vi "pretank.vi"() -> ()   [LabVIEW 2018]
panel:
  in  "stop":bool
  out "Running":bool
  out "String":string
  out "Cup\nFilling":bool
  out "Heater":bool
  out "Belt":bool
  out "Pump":bool
  out "Temperture":dbl(slide) scale=0.0..100.0
  out "TANK":dbl(slide) scale=0.0..10.0
  in  "Temp preset Value":dbl
  in  "Tank Preset Value":dbl
  in  "Heat Tank":dbl
  in  "Fill Tank":dbl
  in  "Reset":bool
  in  "Sensor 2":bool
  in  "Sensor 1":bool
  in  "Start":bool
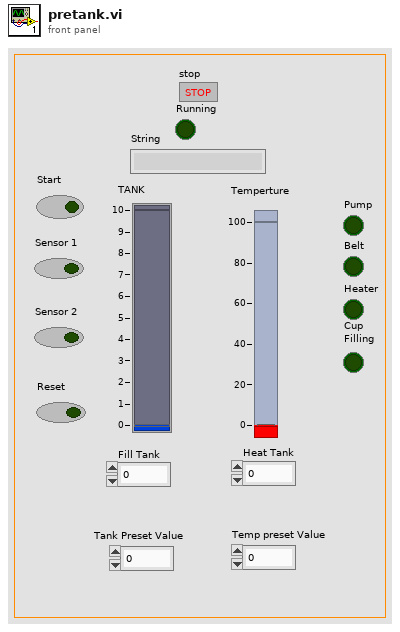
[diagram p1: front panel]
types:
  T1 = enum16{"Start", "Fill", "Sensor 1", "Heat", "Cup", "Sensor 2", "OFF"}
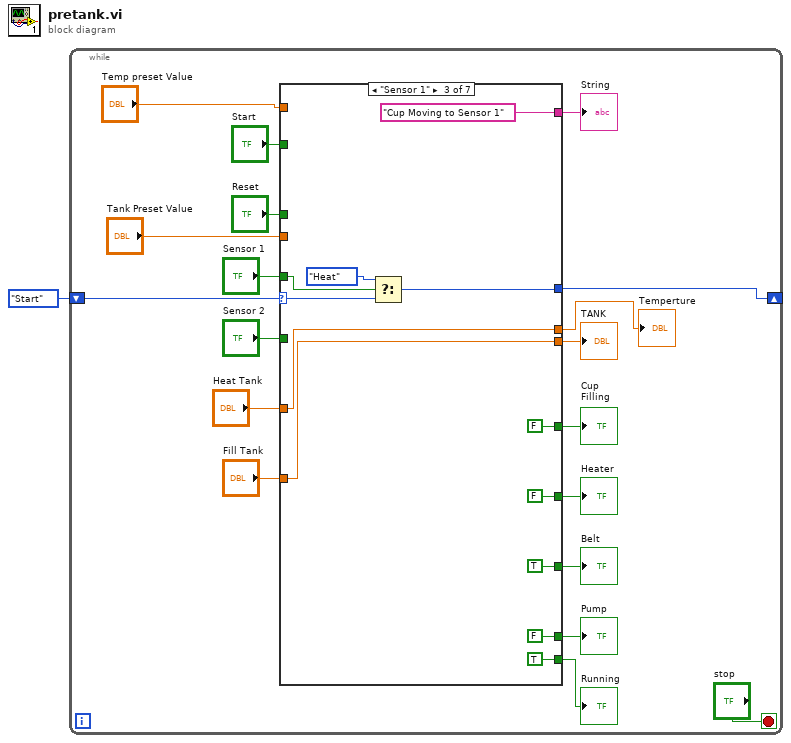
[diagram p0: block diagram]
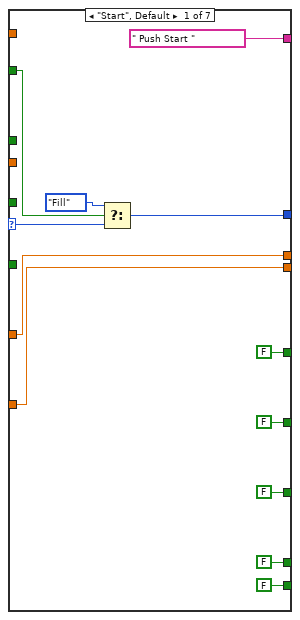
[diagram p2: hidden frame]
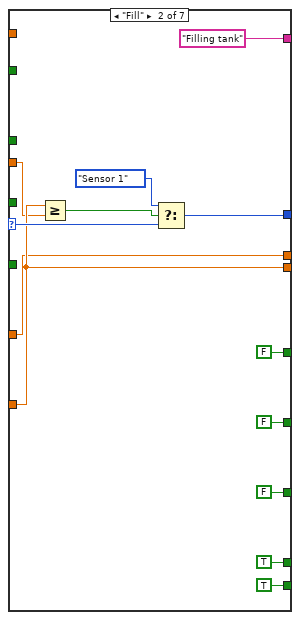
[diagram p3: hidden frame]
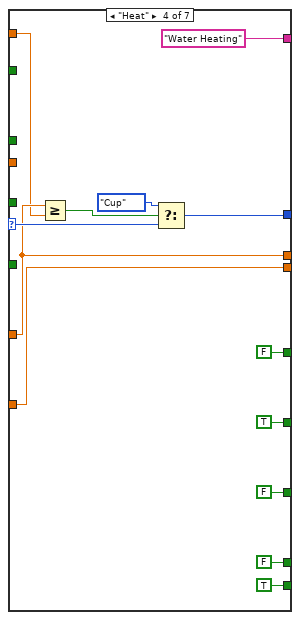
[diagram p4: hidden frame]
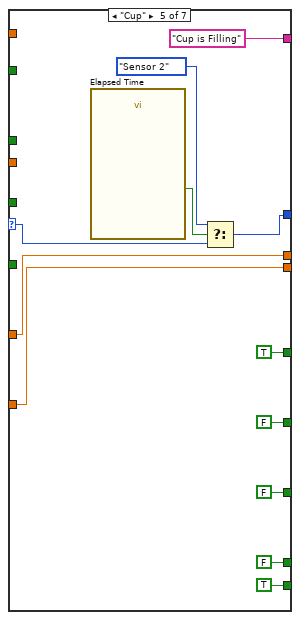
[diagram p5: hidden frame]
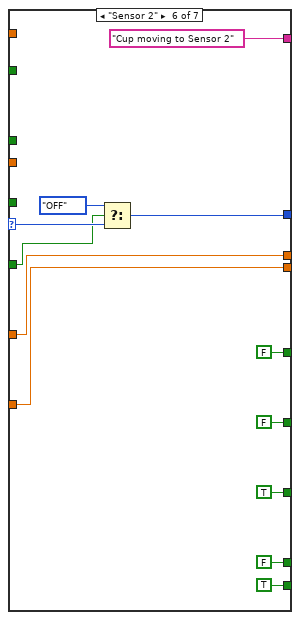
[diagram p6: hidden frame]
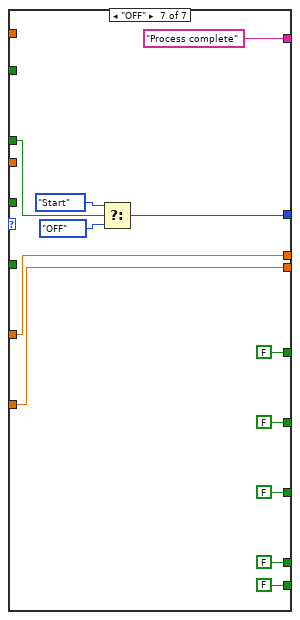
[diagram p7: hidden frame]
diagram:
  n1 = while {
    shift-right: [w12] -> _
    shift-left: T1."Start" -> [w20]
    stop <- "stop" stop-if-true
    n2 = case shown="\"Sensor 1\"" w20 {
      selector: w20 -> [w23 w40 w51 w61 w77 w89 _]
      tunnel: [FALSE FALSE FALSE FALSE TRUE FALSE FALSE] -> w19
      tunnel: [FALSE FALSE FALSE TRUE FALSE FALSE FALSE] -> w18
      tunnel: [FALSE FALSE TRUE FALSE FALSE TRUE FALSE] -> w17
      tunnel: [FALSE TRUE FALSE FALSE FALSE FALSE FALSE] -> w16
      tunnel: [FALSE TRUE TRUE TRUE TRUE TRUE FALSE] -> w15
      tunnel: [" Push Start " "Filling tank" "Cup Moving to Sensor 1" "Water Heating" "Cup is Filling" "Cup moving to Sensor 2" "Process complete"] -> w14
      tunnel: "Reset" -> [_ _ _ _ _ _ w98]
      tunnel: [w25 w41 w49 w64 w78 w91 w97] -> w12
      tunnel: "Start" -> [w24 _ _ _ _ _ _]
      tunnel: [w22 w39 w48 w58 w76 w90 w96] -> w10
      tunnel: "Fill Tank" -> [w22 w39 w48 w58 w76 w90 w96]
      tunnel: [w21 w38 w47 w60 w75 w83 w95] -> w8
      tunnel: "Heat Tank" -> [w21 w38 w47 w60 w75 w83 w95]
      tunnel: "Sensor 1" -> [_ _ w52 _ _ _ _]
      tunnel: "Sensor 2" -> [_ _ _ _ _ w88 _]
      tunnel: "Temp preset Value" -> [_ _ _ w59 _ _ _]
      tunnel: "Tank Preset Value" -> [_ w33 _ _ _ _ _]
      frame "Start", Default {
        n3 = Select(t=T1."Fill", s=w24, f=w23) -> (s? t:f=w25:T1)
      }
      frame "Fill" {
        n4 = Greater Or Equal?(x=w39, y=w33) -> (x >= y?=w44:bool)
        n5 = Select(t=T1."Sensor 1", s=w44, f=w40) -> (s? t:f=w41:T1)
      }
      frame "Sensor 1" {
        n6 = Select(t=T1."Heat", s=w52, f=w51) -> (s? t:f=w49:T1)
      }
      frame "Heat" {
        n7 = Greater Or Equal?(x=w60, y=w59) -> (x >= y?=w62:bool)
        n8 = Select(t=T1."Cup", s=w62, f=w61) -> (s? t:f=w64:T1)
      }
      frame "Cup" {
        n9 = call "Elapsed Time"() -> ("Time has Elapsed"=w81:bool)  [unwired: 12 in, 7 out]
        n10 = Select(t=T1."Sensor 2", s=w81, f=w77) -> (s? t:f=w78:T1)
      }
      frame "Sensor 2" {
        n11 = Select(t=T1."OFF", s=w88, f=w89) -> (s? t:f=w91:T1)
      }
      frame "OFF" {
        n12 = Select(t=T1."Start", s=w98, f=T1."OFF") -> (s? t:f=w97:T1)
      }
    }
    "TANK" <- w10
    "Temperture" <- w8
    "Pump" <- w16
    "Belt" <- w17
    "Heater" <- w18
    "Cup\nFilling" <- w19
    "String" <- w14
    "Running" <- w15
  }
